vi "Object To String.vi"(6 "pretty print? (T)":bool=TRUE, 7 "enable LabVIEW extensions? (T)":bool=TRUE, 8 "error in (no error)":errorcluster, 11 "JSON Value in":refnum<class "JSON Value.lvclass">) -> (0 "error out":errorcluster, 3 "String":string)   [LabVIEW 2016, in "JSON Value.lvclass"]
doc: "Flattens the given JSON data to a string."
uses:
  JSON Value.lvclass
  JSON Value.lvclass/JSON Value.ctl
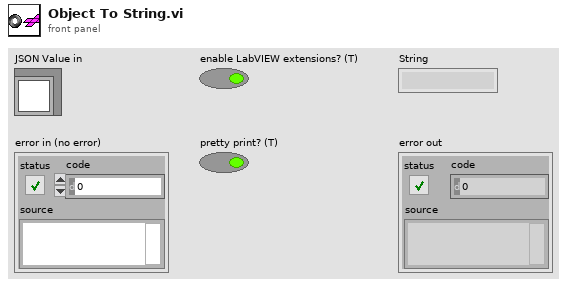
[diagram p1: front panel]
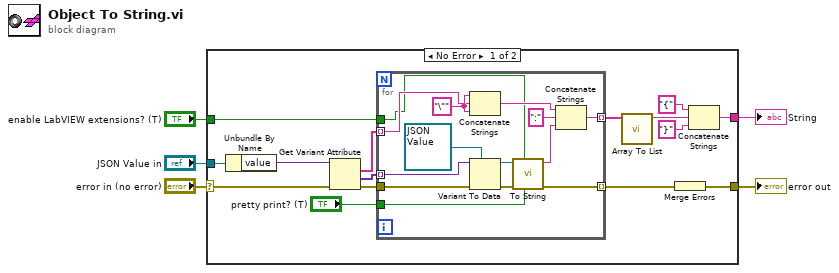
[diagram p0: block diagram]
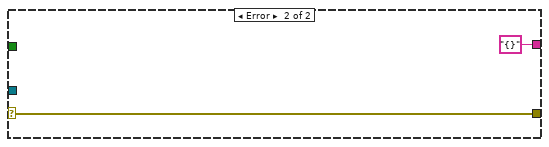
[diagram p2: hidden frame]
diagram:
  n1 = case shown="No Error" "error in (no error)" {
    selector: "error in (no error)" -> [w13 w35]
    tunnel: "JSON Value in" -> [w20 _]
    tunnel: [w16 "{}"] -> w4
    tunnel: [w10 w35] -> w2
    tunnel: "enable LabVIEW extensions? (T)" -> [w7 _]
    frame No Error {
      n2 = Unbundle By Name(w20) -> ("value"=w19:variant)
      n3 = Get Variant Attribute(Variant=w19, error in=w13) -> (names=w18:string[], values=w17:variant[], error out=w12:errorcluster)  [unwired: 2 in, 1 out]
      n4 = for {
        tunnel: w18 -> [w30] mode=indexing
        tunnel: w17 -> [w34] mode=indexing
        tunnel: [w32] -> w15 mode=indexing
        tunnel: w12 -> [w26]
        tunnel: [w24] -> w11 mode=indexing
        tunnel: w7 -> [w23]
        tunnel: "pretty print? (T)" -> [w21]
        w31 = "\"" ("string")
        n5 = Concatenate Strings(w31, w30, w31) -> (w29:string)
        n6 = Variant To Data(error in=w26, type=refnum<class "JSON Value.lvclass"> refnum ("JSON Object in"), Variant=w34) -> (data=w28:refnum<class "JSON Value.lvclass">, error out=w25:errorcluster)
        n7 = call "To String.vi"("pretty print? (T)"=w21, "enable LabVIEW extensions? (T)"=w23, "error in (no error)"=w25, "JSON Value in"=w28) -> ("error out"=w24:errorcluster, "String"=w27:string)  [unwired: 6 in]
        n8 = Concatenate Strings(w29, ":" ("string"), w27) -> (w32:string)
      }
      n9 = call "Array To List.vi"("Array"=w15) -> ("String"=w14:string)  [unwired: 10 in]
      n10 = Merge Errors(w11) -> (w10:errorcluster)
      n11 = Concatenate Strings("{" ("string"), w14, "}" ("string")) -> (w16:string)
    }
    frame Error {
    }
  }
  "String" <- w4
  "error out" <- w2
